vi "test_pathArray.vi"(8 "error in (no error)":errorcluster) -> (0 "error out":errorcluster)   [LabVIEW 2020]
uses:
  run-tests/Run Test (Array Path).vi
  Caraya.lvlib
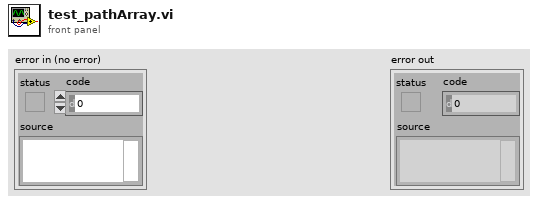
[diagram p1: front panel]
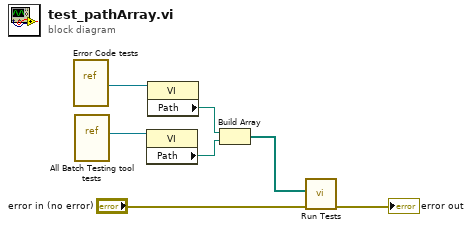
[diagram p0: block diagram]
diagram:
  n1 = vi-ref "Error Code tests.vi"() -> (w7:refnum<vi>)
  n2 = vi-ref "All Batch Testing tool tests.vi"() -> (w4:refnum<vi>)
  n3 = property class="VI"(reference=w4) -> ("Path"=w3:path)  [unwired: 1 in, 2 out]
  n4 = property class="VI"(reference=w7) -> ("Path"=w2:path)  [unwired: 1 in, 2 out]
  n5 = Build Array(w2, w3) -> (w1:path[])
  n6 = call-poly "Run Tests.vi"("error in"="error in (no error)", "Paths"=w1) -> ("error out"=→"error out":errorcluster)  [unwired: 8 in, 1 out]
